vi "PQ Test Time Conversion.vi"(8 "error in (no error)":errorcluster) -> (0 "error out":errorcluster)   [LabVIEW 2019]
uses:
  <vilib>/addons/_JKI Toolkits/Caraya/classes/Assert/Assert.lvclass
  <vilib>/addons/_JKI Toolkits/Caraya/classes/Test/Test.lvclass
  src/LV-Data.PG/LV-Data.PGSQL.lvclass
  src/LV-Data.PG/Typedefs/Time.Datatype--enum.ctl
  <vilib>/addons/_JKI Toolkits/Caraya/classes/Assert/Assert True.vi
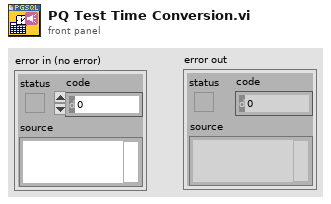
[diagram p1: front panel]
types:
  T1 = typedef "LV-Data.PGSQL.lvclass/Time.Datatype--enum.ctl" = enum16{"timestamp without time zone", "timestamp with time zone"}
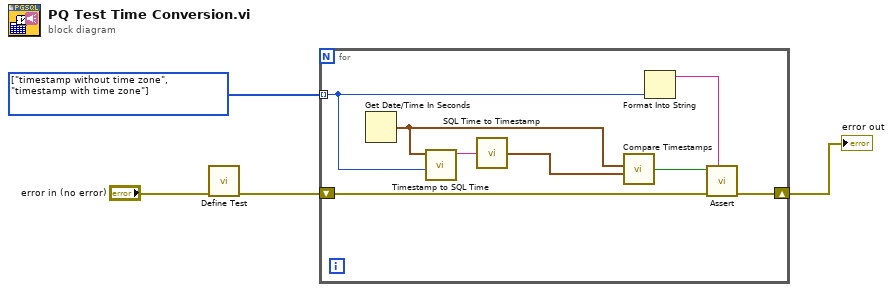
[diagram p0: block diagram]
diagram:
  w1 = T1[] [enum."timestamp without time zone", enum."timestamp with time zone"] items=["timestamp without time zone", "timestamp with time zone"] ("Array")
  n1 = call <vilib>:"Define Test.vi"("error in (no error)"="error in (no error)") -> ("error out"=w2:errorcluster)  [unwired: 9 in, 1 out]
  n2 = for {
    tunnel: w1 -> [w5] mode=indexing
    shift-right: [w12] -> w4
    shift-left: w2 -> [w11]
    n3 = Get Date/Time In Seconds() -> (seconds since 1Jan1904=w9:timestamp)
    n4 = call "Timestamp to SQL Time.vi"("Time Datatype"=w5, "Timestamp"=w9) -> ("date/time string"=w10:string)  [unwired: 9 in]
    n5 = call "SQL Time to Timestamp.vi"("Get:Get String"=w10) -> ("Time Stamp"=w8:timestamp)
    n6 = call <vilib>:"Compare Timestamps.vi"("timestamp (1)"=w9, "timestamp (2)"=w8) -> ("Equal?"=w7:bool)  [unwired: 6 in]
    n7 = Format Into String(w5) -> (resulting string=w6:string)  [unwired: 3 in, 1 out]
    n8 = call-poly <vilib>:"Assert.vi"("Label"=w6, "error in (no error)"=w11, "True?"=w7) -> ("error out"=w12:errorcluster)  [unwired: 7 in, 1 out]
  }
  "error out" <- w4
